vi "Change Panel.vi"(6 "timeout in ms (-1)":i32=-1, 8 "error in (no error)":errorcluster, 10 "New Panel":refnum<class "Panel.lvclass">) -> (0 "error out":errorcluster)   [LabVIEW 2024, in "Anode.lvlib"]
doc: "Changes the Panel type.\n_____\nCreated using Delacor QMH Event Scripter 3.1.0.29.\n\n<b>Note:</b> This VI was modified by the <b>Validate DQMH Module</b> tool to be shared clone reentrant."
uses:
  Anode.lvlib
  <vilib>/MGI/Panel Manager/Panel/Panel/Panel.lvclass
  Change Panel Argument--cluster.ctl
  <vilib>/MGI/Panel Manager/Panel/Panel/Panel.lvclass/Panel.ctl
  <vilib>/MGI/Panel Manager/Panel/Init Waiter/Init Waiter.vi
  <vilib>/MGI/Panel Manager/Panel/Init Waiter/Init Waiter.lvclass
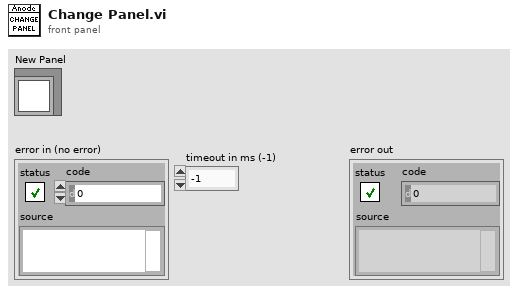
[diagram p1: front panel]
types:
  T1 = typedef "Anode.lvlib/Change Panel Argument--cluster.ctl" = cluster{"New Panel":refnum<class "Panel.lvclass">}
  T2 = typedef "Anode.lvlib/Request Events--cluster.ctl" = cluster{"Stop Module":refnum<user-event>, "Show Panel":refnum<user-event>, "Hide Panel":refnum<user-event>, "Get Module Execution Status":refnum<user-event>, "Show Diagram":refnum<user-event>, "Change Panel":refnum<user-event>, "Set Anode Inlet Pressure SP":refnum<user-event>, "Initialise Pressure Regulator Interface":refnum<user-event>, "Start Polling Pressure Regulator Status":refnum<user-event>, "Stop Polling Pressure Regulator Status":refnum<user-event>, "Read Pressure Regulator Status":refnum<user-event>, "Set Pressure Regulator Control Function":refnum<user-event>, "Set Anode Inlet Flow SP":refnum<user-event>, "Set Anode Inlet Valve State":refnum<user-event>, "Private":cluster{"Wake Connection Helper Loop":refnum<user-event>}, "Set Anode Gas Supply Valve":refnum<user-event>, "Set Purge Valve":refnum<user-event>, "Set Purge Strategy":refnum<user-event>, "Private.Wake Purge Strategy Helper Loop":refnum<user-event>, "Private.Update Purge Strategy Settings":refnum<user-event>, "Wake Purge Helper Loop":refnum<user-event>, "Wake Recirculation Pump Helper Loop":refnum<user-event>, "Sleep Recirculation Pump Helper Loop":refnum<user-event>, "Set Pump Speed SP":refnum<user-event>, "Set Pump Enable State":refnum<user-event>, "Set Pump Speed Control Mode":refnum<user-event>, "Private.Update Purge Strategy Helper Loop":refnum<user-event>, "Force Purge":refnum<user-event>, "Reset Counter":refnum<user-event>, "Private.Wake H2 Sensor Loop":refnum<user-event>, "Private.Sleep H2 Sensor Loop":refnum<user-event>, "Start H2 Sensor Measurement":refnum<user-event>, "Stop H2 Sensor Measurement":refnum<user-event>}
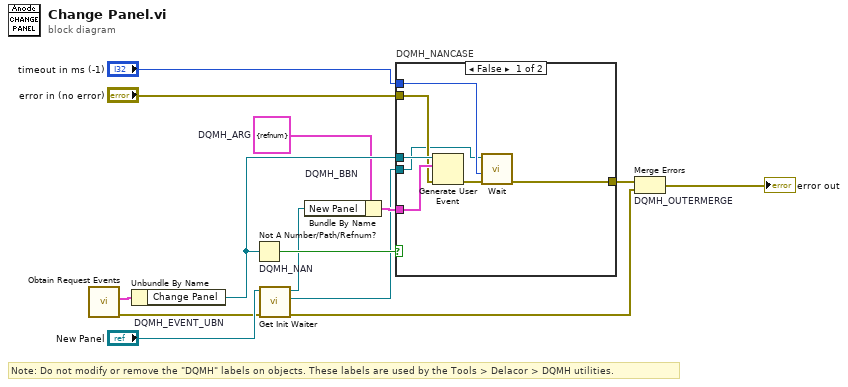
[diagram p0: block diagram]
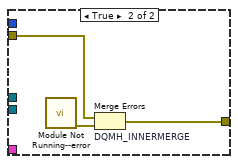
[diagram p2: hidden frame]
diagram:
  w8 = T1 {"New Panel"=refnum}  # DQMH_ARG
  # "Note: Do not modify or remove the \"DQMH\" labels on objects. These labels are used by the Tools > Delacor > DQMH utilities."
  n1 = call "Obtain Request Events.vi"() -> ("error out"=w3:errorcluster, "Anode Request Events"=w7:T2)  [unwired: 10 in]
  n2 = Unbundle By Name "DQMH_EVENT_UBN"(w7) -> ("Change Panel"=w10:refnum<user-event>)
  n3 = Not A Number/Path/Refnum? "DQMH_NAN"(number/path/refnum=w10) -> (NaN/Path/Refnum?=w11:bool)
  n4 = call <vilib>:"Get Init Waiter.vi"("Error In"=w3, "Panel In"="New Panel") -> ("Error Out"=w2:errorcluster, "Init Waiter"=w1:refnum<class "Init Waiter.lvclass">, "Panel Out"=w4:refnum<class "Panel.lvclass">)  [unwired: 7 in]
  n5 = Bundle By Name "DQMH_BBN"(cluster=w8, "New Panel"=w4) -> (w12:T1)
  n6 = case "DQMH_NANCASE" shown="False" w11 {
    tunnel: "error in (no error)" -> [w19 w24]
    tunnel: [w17 w23] -> w9
    tunnel: w10 -> [w21 _]
    tunnel: w12 -> [w20 _]
    tunnel: "timeout in ms (-1)" -> [w16 _]
    tunnel: w1 -> [w15 _]
    frame False {
      n7 = Generate User Event(user event=w21, event data cluster=w20, error in=w19) -> (error out=w18:errorcluster)  [unwired: 1 in, 1 out]
      n8 = call <vilib>:"Wait.vi"("Error In"=w18, "timeout in ms (-1)"=w16, "Init Waiter in"=w15) -> ("Error Out"=w17:errorcluster)  [unwired: 7 in, 1 out]
    }
    frame True {
      n9 = call "Module Not Running--error.vi"() -> ("error out"=w22:errorcluster)  [unwired: 11 in]
      n10 = Merge Errors "DQMH_INNERMERGE"(w24, w22) -> (w23:errorcluster)
    }
  }
  n11 = Merge Errors "DQMH_OUTERMERGE"(w9, w2) -> (→"error out":errorcluster)
